vi "Assisted Turning.vi"(2 "Left":bool=TRUE, 3 "Current Value":dbl format="%#_13g", 4 "Right":bool, 5 "Turn Amount":dbl=90.0 format="%#_13g") -> (0 "New Value":dbl format="%#_13g", 1 "Same Target":bool)   [LabVIEW 2016]
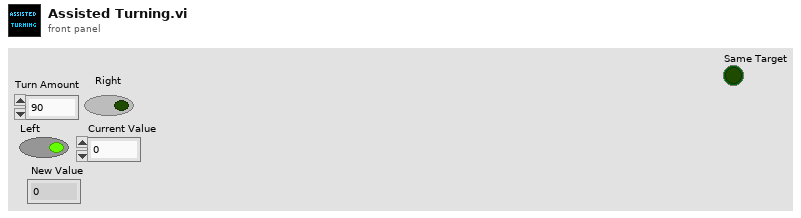
[diagram p1: front panel]
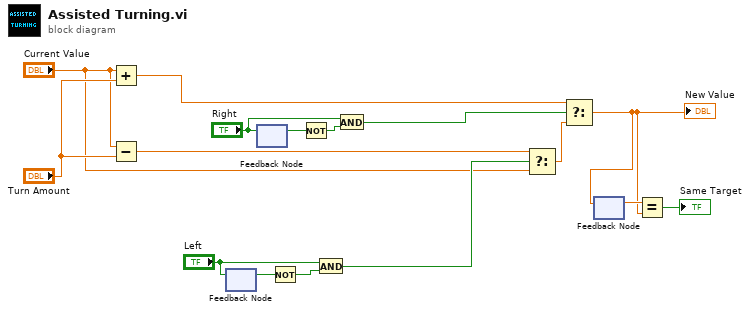
[diagram p0: block diagram]
diagram:
  n1 = Add(x="Current Value", y="Turn Amount") -> (x+y=w5:dbl)
  n2 = Subtract(x="Current Value", y="Turn Amount") -> (x-y=w6:dbl)
  n3 = feedback-in #1("Left") -> ()
  n4 = feedback #1() -> (w15:bool)  [unwired: 1 in]
  n5 = feedback-in #2("Right") -> ()
  n6 = feedback #2() -> (w11:bool)  [unwired: 1 in]
  n7 = Not(x=w15) -> (.not. x?=w14:bool)
  n8 = Not(x=w11) -> (.not. x?=w12:bool)
  n9 = And(x="Left", y=w14) -> (x .and. y?=w9:bool)
  n10 = And(x="Right", y=w12) -> (x .and. y?=w8:bool)
  n11 = Select(t=w6, s=w9, f="Current Value") -> (s? t:f=w10:dbl)
  n12 = Select(t=w5, s=w8, f=w10) -> (s? t:f=w2:dbl)
  "New Value" <- w2
  n13 = feedback-in #3(w2) -> ()
  n14 = feedback #3() -> (w3:dbl)  [unwired: 1 in]
  n15 = Equal?(x=w3, y=w2) -> (x = y?=→"Same Target":bool)
